vi "Pre Launch Init.vi"(11 "Controller in":refnum<class "Controller.lvclass">) -> (0 "error out":errorcluster, 3 "Controller out":refnum<class "Controller.lvclass">)   [LabVIEW 2018, in "Controller.lvlib" / "Controller.lvclass"]
doc: "The <b>Controller::Pre Launch Init</b> reads data from the configuration file concerning the"
uses:
  Controller.lvclass
  <vilib>/ActorFramework/Actor/Actor.lvclass
  Controls/Notifier Enum.ctl
  <vilib>/Utility/config.llb/NI_LVConfig.lvlib
  <vilib>/Utility/config.llb/Read Key (Boolean).vi
  <vilib>/Utility/config.llb/Read Key (I32).vi
  reusable/Switch/Switch.lvclass
  <vilib>/NI_Real-Time Target Support.lvlib
  Messages/Update Filter State Params/Update Filter Cycle Params MSG.lvclass
  Messages/Change Filter State/Change Filter State.lvclass
  <vilib>/ActorFramework/Message Enqueuer/Message Enqueuer.lvclass
  Messages/Change Inlet MSG/Change Inlet MSG.lvclass
  SuperActor/SuperActor.lvclass
  Messages/O3 Valve MSG/O3 Valve MSG.lvclass
  reusable/Session APIs/CVT/CVT.lvclass
  Messages/Change Denuder State/Change Denuder State MSG.lvclass
  C:/Users/Labview/Documents/exscalabar_server/SuperActor/SuperActor.lvclass
  C:/Program Files (x86)/National Instruments/LabVIEW 2018/vi.lib/ActorFramework/Actor/Actor.lvclass
  <userlib>/_Session Fwk/Session - Root.lvclass
  C:/Users/Labview/Documents/exscalabar_server/Controller/Messages/Update Switch State MSG/Update Switch MSG.lvclass
  C:/Program Files (x86)/National Instruments/LabVIEW 2018/vi.lib/ActorFramework/Message/Message.lvclass
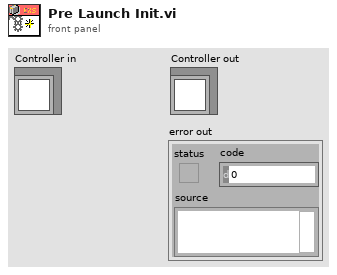
[diagram p1: front panel]
types:
  T1 = typedef "Controller.lvlib/Controller.lvclass/Notifier Enum.ctl" = enum16{"Initialize", "Get", "Set", "Close"}
  T2 = typedef "Session - Root.lvclass/Session Handle.ctl" = refnum<data-value>
  T3 = typedef "NI_LVConfig.lvlib/Config Data RefNum.ctl" = refnum<k1>
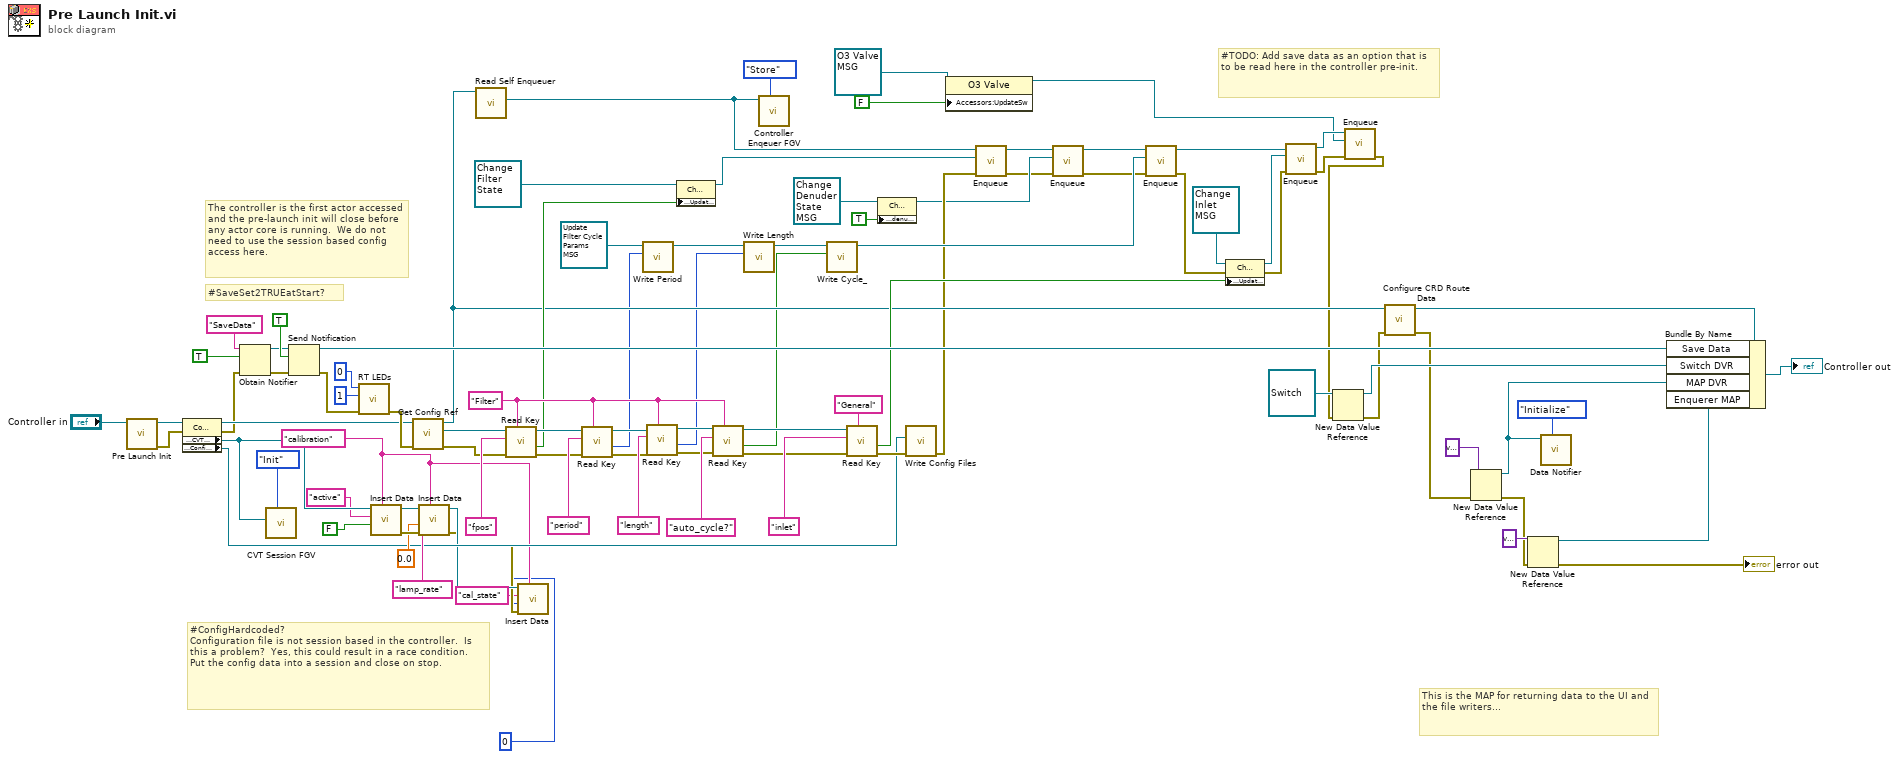
[diagram p0: block diagram]
diagram:
  w10 = "calibration" ("Group")
  w84 = "Filter" ("section")
  # "This is the MAP for returning data to the UI and the file writers..."
  # "#ConfigHardcoded?\nConfiguration file is not session based in the controller.  Is this a problem?  Yes, this could result in a race condition.  Put the config data into a session and close on stop."
  # "#SaveSet2TRUEatStart?"
  # "The controller is the first actor accessed and the pre-launch init will close before any actor core is running.  We do not need to use the session based config access here."
  # "#TODO: Add save data as an option that is to be read here in the controller pre-init."
  n1 = call-parent "Pre Launch Init.vi"("Ex Nested in"="Controller in") -> ("error out"=w43:errorcluster, "Ex Nested out"=w46:refnum<class "Controller.lvclass">)  [unwired: 9 in]
  n2 = property class="Controller"(reference=w46, error in=w43) -> (reference out=w44:refnum<class "Controller.lvclass">, error out=w42:errorcluster, "Accessors:CVT Session"=w29:T2, "Accessors:Config Session"=w13:T2)
  n3 = Obtain Notifier(name (unnamed)="SaveData", notification data type=TRUE, error in (no error)=w42) -> (notifier out=w68:refnum<notifier>, error out=w69:errorcluster)  [unwired: 1 in, 1 out]
  n4 = call "CVT Session FGV.vi"("State"=enum16{"Init", "Get"}."Init", "CVT Session"=w29) -> ()  [unwired: 9 in, 1 out]
  n5 = Send Notification(notification=TRUE, notifier=w68, error in (no error)=w69) -> (notifier out=w71:refnum<notifier>, error out=w49:errorcluster)
  n6 = call <vilib>:"RT LEDs.vi"("error in (no error)"=w49, "State"=1, "LED Num"=0) -> ("error out"=w53:errorcluster)  [unwired: 3 in, 1 out]
  n7 = call "Insert Data.vi"("Group"=w10, "Data"=FALSE, "tag"="active", "CVT Session In"=w29) -> ("error out"=w19:errorcluster, "CVT Session Out"=w18:T2)  [unwired: 6 in]
  n8 = call "Get Config Ref.vi"("error in"=w53, "Ex Nested in"=w44) -> ("error out"=w52:errorcluster, "config ref"=w51:T3, "Ex Nested out"=w50:refnum<class "Controller.lvclass">)  [unwired: 7 in]
  n9 = call "Insert Data.vi"("Group"=w10, "error in"=w19, "Data"=0.0, "tag"="lamp_rate", "CVT Session In"=w18) -> ("error out"=w11:errorcluster, "CVT Session Out"=w12:T2)  [unwired: 5 in]
  n10 = call <vilib>:"Read Self Enqueuer.vi"("Actor"=w50) -> ("Self Enqueuer"=w87:refnum<class "Message Enqueuer.lvclass">)  [unwired: 10 in]
  n11 = call-poly <vilib>:"Read Key.vi"("section"=w84, "error in (no error)"=w52, "key"="fpos", "refnum"=w51) -> ("error out"=w74:errorcluster, "value"=w63:bool, "refnum out"=w73:T3)  [unwired: 4 in, 1 out]
  n12 = call "Insert Data.vi"("Group"=w10, "error in"=w11, "Data"=u8 0, "tag"="cal_state", "CVT Session In"=w12) -> ()  [unwired: 5 in, 2 out]
  n13 = call-poly <vilib>:"Read Key.vi"("section"=w84, "error in (no error)"=w74, "key"="period", "refnum"=w73) -> ("error out"=w77:errorcluster, "value"=w24:i32, "refnum out"=w76:T3)  [unwired: 4 in, 1 out]
  n14 = call "Write Period.vi"("Period"=w24, "Update Filter Cycle Params MSG in"=refnum<class "Update Filter Cycle Params MSG.lvclass"> refnum ("Controller.lvlib:Update Filter Cycle Params")) -> ("Update Filter Cycle Params MSG out"=w22:refnum<class "Update Filter Cycle Params MSG.lvclass">)  [unwired: 8 in, 1 out]
  n15 = call-poly <vilib>:"Read Key.vi"("section"=w84, "error in (no error)"=w77, "key"="length", "refnum"=w76) -> ("error out"=w83:errorcluster, "value"=w23:i32, "refnum out"=w82:T3)  [unwired: 4 in, 1 out]
  n16 = property class="Change Filter State MSG"(reference=refnum<class "Change Filter State.lvclass"> refnum ("Controller.lvlib:Change Filter State MSG"), "Accessors:UpdateSw"=w63) -> (reference out=w61:refnum<class "Change Filter State.lvclass">)  [unwired: 1 in, 1 out]
  n17 = call-poly <vilib>:"Read Key.vi"("section"=w84, "error in (no error)"=w83, "key"="auto_cycle?", "refnum"=w82) -> ("error out"=w48:errorcluster, "value"=w26:bool, "refnum out"=w90:T3)  [unwired: 4 in, 1 out]
  n18 = call "Write Length.vi"("Length"=w23, "Update Filter Cycle Params MSG in"=w22) -> ("Update Filter Cycle Params MSG out"=w21:refnum<class "Update Filter Cycle Params MSG.lvclass">)  [unwired: 8 in, 1 out]
  n19 = call "Controller Enqeuer FGV.vi"("State"=enum16{"Store", "Send MSG"}."Store", "Enqueuer"=w87) -> ()  [unwired: 9 in, 1 out]
  n20 = call "Write Cycle_.vi"("Cycle?"=w26, "Update Filter Cycle Params MSG in"=w21) -> ("Update Filter Cycle Params MSG out"=w20:refnum<class "Update Filter Cycle Params MSG.lvclass">)  [unwired: 8 in, 1 out]
  n21 = call-poly <vilib>:"Read Key.vi"("section"="General", "error in (no error)"=w48, "key"="inlet", "refnum"=w90) -> ("error out"=w15:errorcluster, "value"=w58:bool)  [unwired: 4 in, 2 out]
  n22 = property class="Change Denuder State MSG"(reference=refnum<class "Change Denuder State MSG.lvclass"> refnum ("Controller:Change Denuder State MSG"), "Accessors:denude_"=TRUE ("denude_")) -> (reference out=w5:refnum<class "Change Denuder State MSG.lvclass">)  [unwired: 1 in, 1 out]
  n23 = call "Write Config Files.vi"("error in (no error)"=w15, "Accessors:Config Session"=w13) -> ("error out"=w14:errorcluster)  [unwired: 9 in]
  n24 = property class="O3 Valve"(reference=refnum<class "O3 Valve MSG.lvclass"> refnum ("Controller:O3 Valve"), "Accessors:UpdateSw"=FALSE ("UpdateSw")) -> (reference out=w30:refnum<class "O3 Valve MSG.lvclass">)  [unwired: 1 in, 1 out]
  n25 = call <vilib>:"Enqueue.vi"("error in (no error)"=w14, "Message"=w61, "Message Enqueuer in"=w87) -> ("error out"=w2:errorcluster, "Message Enqueuer out"=w4:refnum<class "Message Enqueuer.lvclass">)  [unwired: 7 in]
  n26 = call <vilib>:"Enqueue.vi"("error in (no error)"=w2, "Message"=w5, "Message Enqueuer in"=w4) -> ("error out"=w1:errorcluster, "Message Enqueuer out"=w3:refnum<class "Message Enqueuer.lvclass">)  [unwired: 7 in]
  n27 = call <vilib>:"Enqueue.vi"("error in (no error)"=w1, "Message"=w20, "Message Enqueuer in"=w3) -> ("error out"=w57:errorcluster, "Message Enqueuer out"=w93:refnum<class "Message Enqueuer.lvclass">)  [unwired: 7 in]
  n28 = property class="Change Inlet MSG.lvclass"(reference=refnum<class "Change Inlet MSG.lvclass"> refnum ("Controller.lvlib:Change Inlet MSG.lvclass"), error in=w57, "Accessors:UpdateSw"=w58) -> (reference out=w59:refnum<class "Change Inlet MSG.lvclass">, error out=w56:errorcluster)
  n29 = call <vilib>:"Enqueue.vi"("error in (no error)"=w56, "Message"=w59, "Message Enqueuer in"=w93) -> ("error out"=w33:errorcluster, "Message Enqueuer out"=w31:refnum<class "Message Enqueuer.lvclass">)  [unwired: 7 in]
  n30 = call <vilib>:"Enqueue.vi"("error in (no error)"=w33, "Message"=w30, "Message Enqueuer in"=w31) -> ("error out"=w32:errorcluster)  [unwired: 7 in, 1 out]
  n31 = New Data Value Reference(data value=refnum<class "Switch.lvclass"> refnum ("Switch"), error in=w32) -> (data value reference=w88:refnum<data-value>, error out=w47:errorcluster)
  n32 = call "Configure CRD Route Data.vi"("error in"=w47, "Controller in"=w50) -> ("error out"=w39:errorcluster, "Controller out"=w54:refnum<class "Controller.lvclass">)  [unwired: 8 in]
  n33 = New Data Value Reference(data value=variant, error in=w39) -> (data value reference=w41:refnum<data-value>, error out=w37:errorcluster)
  n34 = New Data Value Reference(data value=variant, error in=w37) -> (data value reference=w38:refnum<data-value>, error out=→"error out":errorcluster)
  n35 = call "Data Notifier.vi"("State"=Notifier_Enum."Initialize", "MAP DVR"=w41) -> ()  [unwired: 8 in, 2 out]
  n36 = Bundle By Name(cluster=w54, "Save Data"=w71, "Switch DVR"=w88, "MAP DVR"=w41, "Enquerer MAP"=w38) -> (→"Controller out":refnum<class "Controller.lvclass">)
